vi "Send Regular Message.vi"   [LabVIEW 2023, in "Message Handler.lvclass"]
doc: "Set of polymorfic VI that facilitates messaging to processes."
uses:
  Message Handler.lvclass
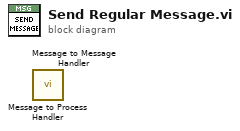
[diagram p0: block diagram]
diagram:
  n1 = call "Message to Process Handler.vi"() -> ()  [unwired: 13 in, 3 out]
  n2 = call "Message to Message Handler.vi"() -> ()  [unwired: 13 in, 3 out]
